vi "split columns.vi"(0 "Display string":string, 11 "error in":errorcluster) -> (4 "start chars":i32[](array[numeric]), 6 "Lengths":i32[](array[numeric]), 8 "Col Headers":string[](array[string]), 10 "Array":string[][](array[string]), 15 "error out":errorcluster)   [LabVIEW 2018]
uses:
  <vilib>/regexp/Match Regular Expression.xnode
panel:
  out "Display string 3":string
  out "Display string 2":string
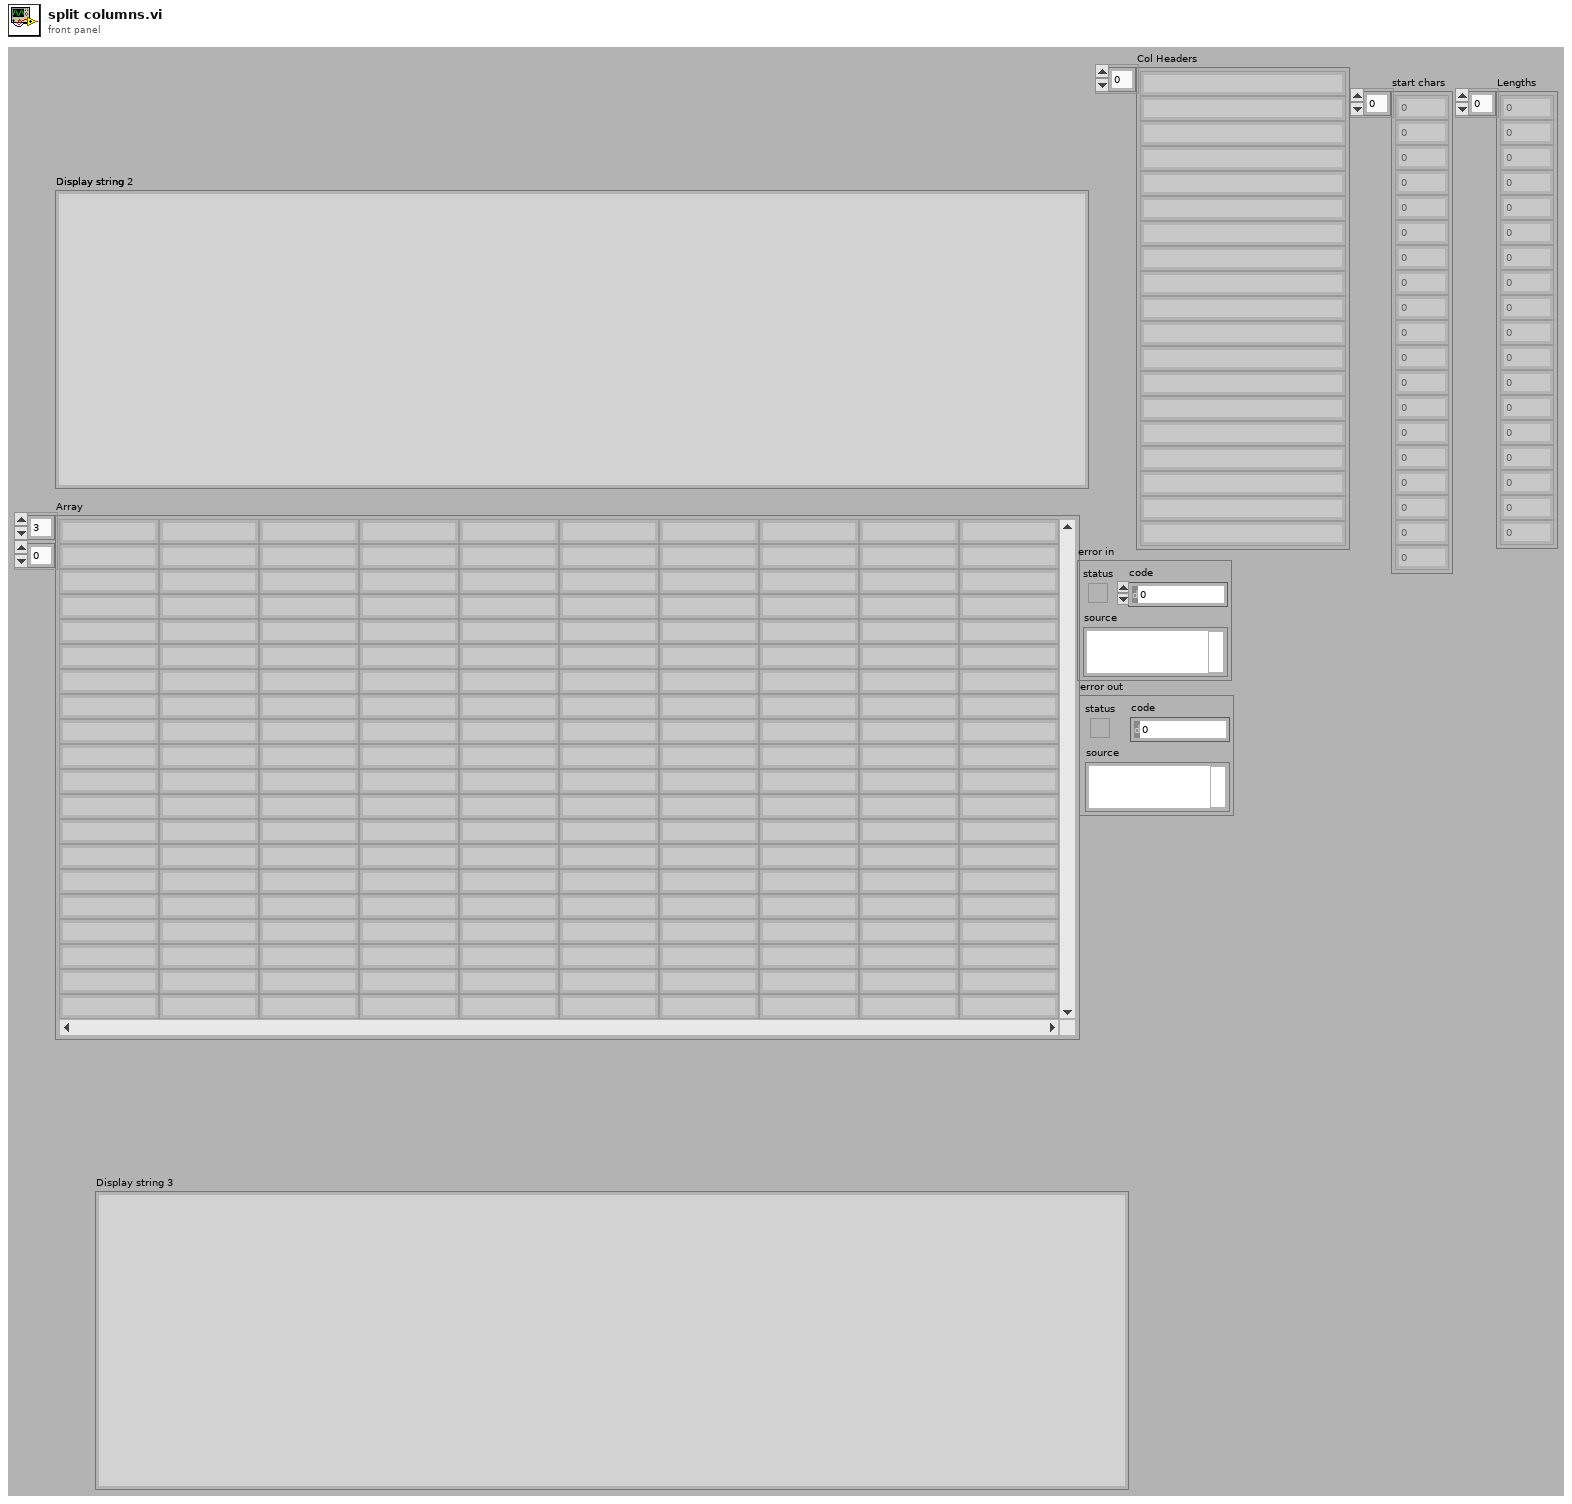
[diagram p1: front panel]
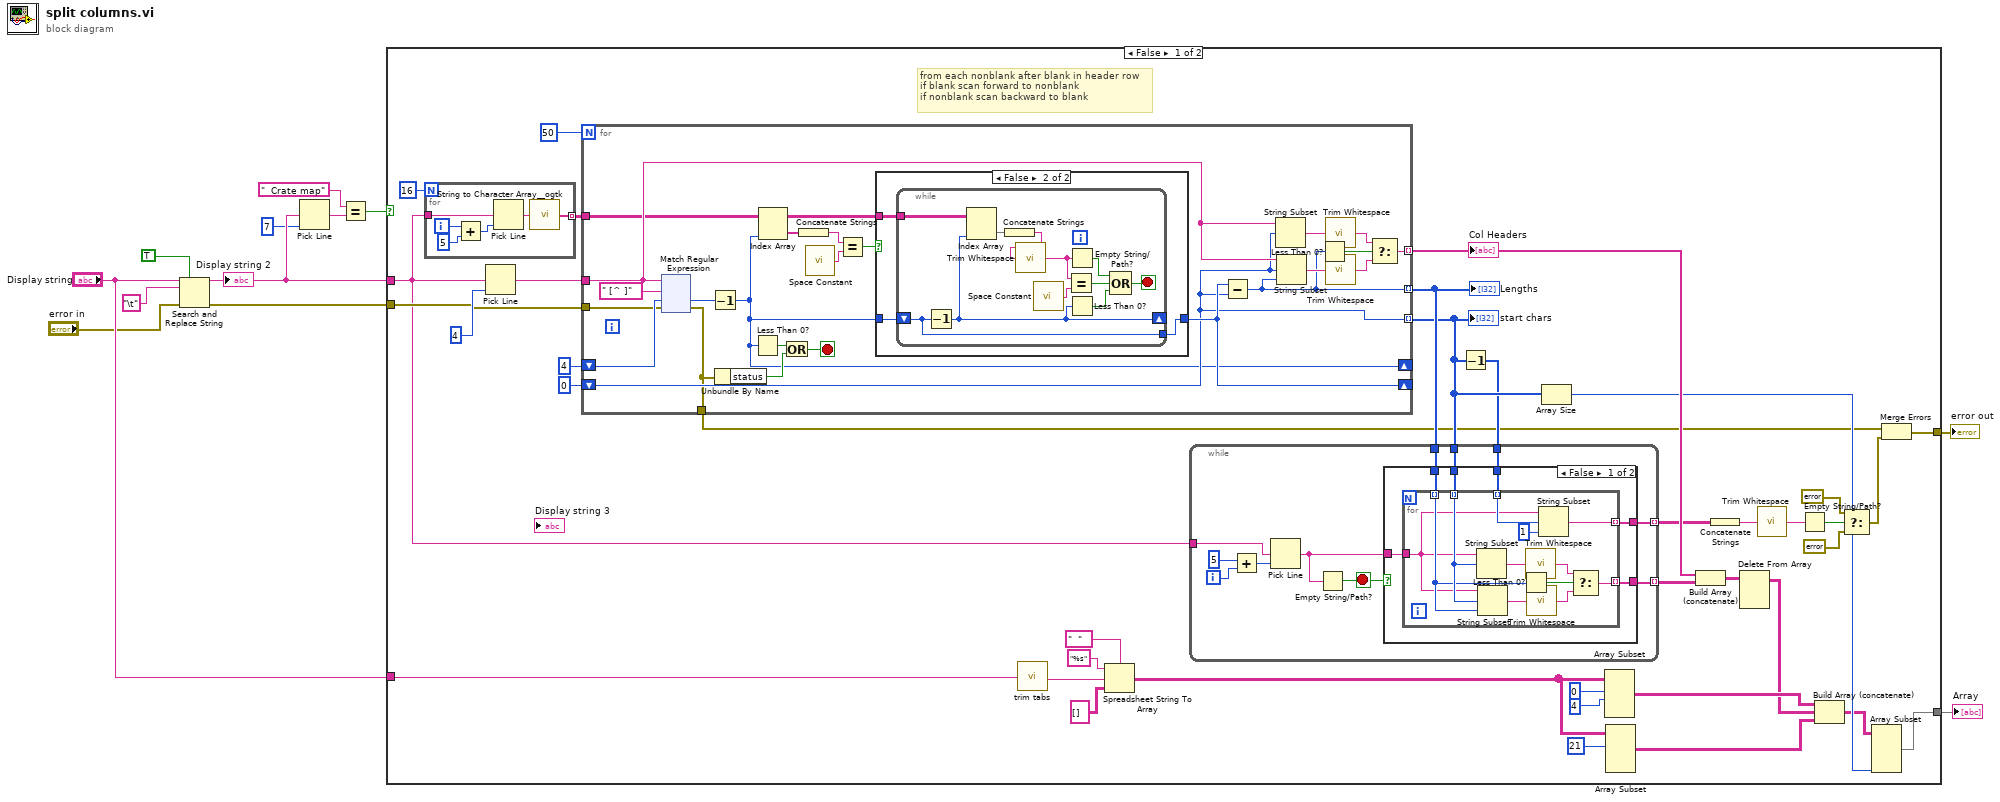
[diagram p0: block diagram]
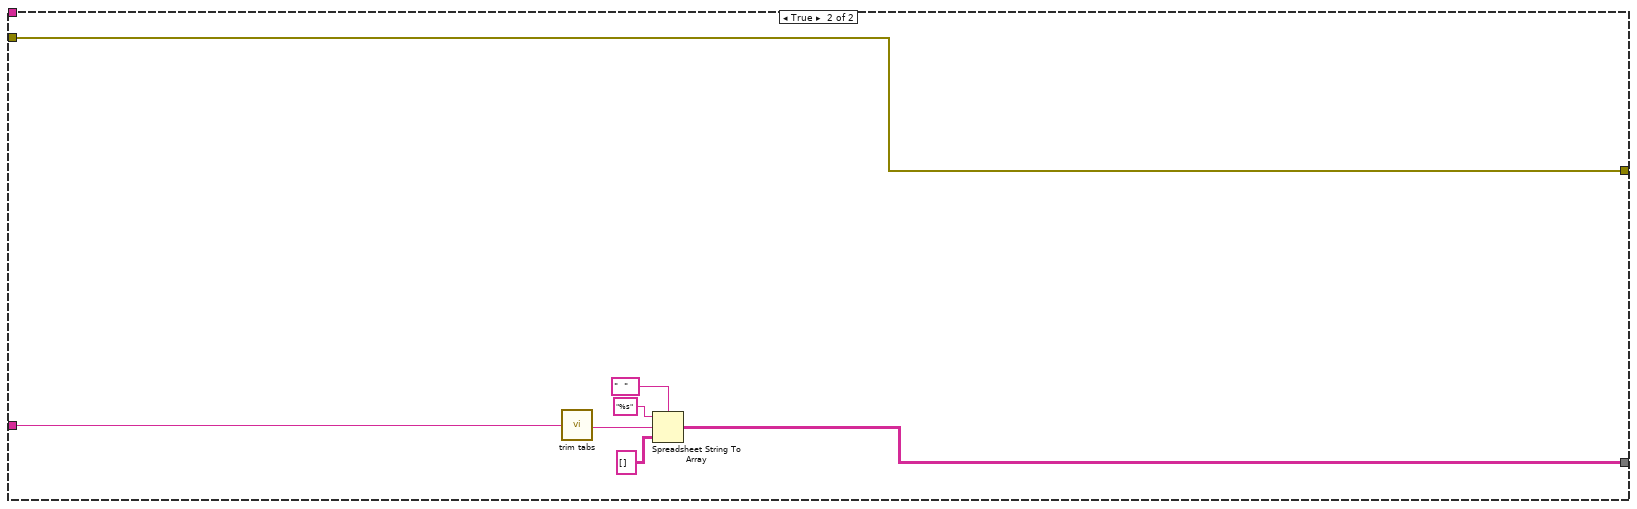
[diagram p4: hidden frame]
diagram:
  n1 = Search and Replace String(replace all?=TRUE ("replace all? (F)"), input string="Display string", search string="\t", error in="error in") -> (result string=w9:string, error out=w2:errorcluster)  [unwired: 4 in, 2 out]
  "Display string 2" <- w9
  n2 = Pick Line(multi-line string=w9, line index=7 ("x")) -> (output string=w7:string)  [unwired: 1 in]
  n3 = Equal?(x="  Crate map" ("search string/char (-)"), y=w7) -> (x = y?=w4:bool)
  n4 = case shown="False" w4 {
    tunnel: "Display string" -> [w43 w239]
    tunnel: w9 -> [w26 _]
    tunnel: [w29 w238] -> w5
    tunnel: w2 -> [w28 w237]
    tunnel: [w14 w237] -> w1
    frame False {
      # "from each nonblank after blank in header row\nif blank scan forward to nonblank\nif nonblank scan backward to blank"
      n5 = for {
        N: 16 -> [_]
        tunnel: w26 -> [w57]
        tunnel: [w52] -> w24 mode=indexing
        i -> [w55]
        n6 = Add(x=w55, y=5 ("x")) -> (x+y=w56:i32)
        n7 = Pick Line(multi-line string=w57, line index=w56) -> (output string=w53:string)  [unwired: 1 in]
        n8 = call <userlib>:"String to Character Array__ogtk.vi"("Input String"=w53) -> ("Character Array"=w52:string[])
      }
      n9 = Pick Line(multi-line string=w26, line index=4 ("x")) -> (output string=w51:string)  [unwired: 1 in]
      n10 = for {
        N: 50 -> [_]
        tunnel: w51 -> [w74]
        shift-right: [w60] -> _
        shift-left: 4 ("x") -> [w76]
        tunnel: [w73] -> w23 mode=indexing
        shift-right: [w78] -> _
        shift-left: 0 ("x") -> [w73]
        tunnel: [w67] -> w47 mode=indexing
        tunnel: [w71] -> w46 mode=indexing
        tunnel: w28 -> [w66]
        tunnel: [w63] -> w13
        tunnel: w24 -> [w61]
        stop <- w62 stop-if-true
        n11 = xnode "Match Regular Expression"("input string"=w74, "regular expression"=" [^ ]" ("search string/char (-)"), "offset (0)"=w76, "error in"=w66) -> ("offset past match"=w77:i32, "error out"=w63:errorcluster)  [unwired: 2 in, 3 out]
        n12 = Decrement(x=w77) -> (x-1=w60:i32)
        n13 = Unbundle By Name(w63) -> ("status"=w65:bool)
        n14 = Less Than 0?(x=w60) -> (x < 0?=w64:bool)
        n15 = Index Array(array=w61, index (col)=w60) -> (element=w59:string[])  [unwired: 1 in]
        n16 = Or(x=w64, y=w65) -> (x .or. y?=w62:bool)
        n17 = Concatenate Strings(w59) -> (w58:string)
        n18 = call <vilib>:"Space Constant.vi"() -> ("String"=w80:string)
        n19 = Equal?(x=w58, y=w80) -> (x = y?=w79:bool)
        n20 = case shown="False" w79 {
          tunnel: w60 -> [w193 w196]
          tunnel: [w193 w195] -> w78
          tunnel: w61 -> [_ w194]
          frame True {
          }
          frame False {
            n21 = while {
              shift-right: [w200] -> _
              shift-left: w196 -> [w206]
              tunnel: [w206] -> w195
              tunnel: w194 -> [w201]
              stop <- w203 stop-if-true
              n22 = Decrement(x=w206) -> (x-1=w200:i32)
              n23 = Index Array(array=w201, index (col)=w200) -> (element=w199:string[])  [unwired: 1 in]
              n24 = Concatenate Strings(w199) -> (w197:string)
              n25 = call <vilib>:"Trim Whitespace.vi"("string"=w197) -> ("trimmed string"=w198:string)  [unwired: 1 in]
              n26 = call <vilib>:"Space Constant.vi"() -> ("String"=w207:string)
              n27 = Equal?(x=w198, y=w207) -> (x = y?=w204:bool)
              n28 = Empty String/Path?(string/path=w198) -> (empty?=w205:bool)
              n29 = Less Than 0?(x=w200) -> (x < 0?=w202:bool)
              n30 = Compound Arithmetic op=OR(w205, w204, w202) -> (w203:bool)
            }
          }
        }
        n31 = Subtract(x=w78, y=w73) -> (x-y=w71:i32)
        n32 = String Subset(string=w74, offset (0)=w73) -> (substring=w72:string)  [unwired: 1 in]
        n33 = String Subset(string=w74, offset (0)=w73, length (rest)=w71) -> (substring=w75:string)
        n34 = Less Than 0?(x=w71) -> (x < 0?=w69:bool)
        n35 = call <vilib>:"Trim Whitespace.vi"("string"=w72) -> ("trimmed string"=w70:string)  [unwired: 1 in]
        n36 = call <vilib>:"Trim Whitespace.vi"("string"=w75) -> ("trimmed string"=w68:string)  [unwired: 1 in]
        n37 = Select(t=w70, s=w69, f=w68) -> (s? t:f=w67:string)
      }
      "Col Headers" <- w47
      "start chars" <- w23
      "Lengths" <- w46
      n38 = call "trim tabs.vi"("string"=w43) -> ("result string"=w42:string)
      n39 = Spreadsheet String To Array(delimiter (Tab)="  ", format string="%s" ("delimiter (Tab)"), spreadsheet string=w42, array type (2D Dbl)=string[][] [] ("appended array")) -> (array=w33:string[][])
      n40 = Decrement(x=w23) -> (x-1=w22:i32[])
      n41 = while {
        tunnel: w26 -> [w215]
        tunnel: w23 -> [w214]
        tunnel: w46 -> [w213]
        tunnel: [w212] -> w45 mode=indexing
        tunnel: w22 -> [w209]
        tunnel: [w208] -> w21 mode=indexing
        i -> [w216]
        stop <- w210 stop-if-true
        n42 = Add(x=5, y=w216) -> (x+y=w218:i32)
        n43 = Pick Line(multi-line string=w215, line index=w218) -> (output string=w211:string)  [unwired: 1 in]
        n44 = Empty String/Path?(string/path=w211) -> (empty?=w210:bool)
        n45 = case shown="False" w210 {
          tunnel: w214 -> [w224 _]
          tunnel: w213 -> [w223 _]
          tunnel: [w222 _] -> w212
          tunnel: w211 -> [w221 _]
          tunnel: w209 -> [w220 _]
          tunnel: [w219 _] -> w208
          frame False {
            n46 = for {
              tunnel: w221 -> [w226]
              tunnel: w224 -> [w230] mode=indexing
              tunnel: w223 -> [w229] mode=indexing
              tunnel: [w231] -> w222 mode=indexing
              tunnel: w220 -> [w228] mode=indexing
              tunnel: [w225] -> w219 mode=indexing
              n47 = String Subset(string=w226, offset (0)=w230) -> (substring=w233:string)  [unwired: 1 in]
              n48 = String Subset(string=w226, offset (0)=w230, length (rest)=w229) -> (substring=w232:string)
              n49 = Less Than 0?(x=w229) -> (x < 0?=w235:bool)
              n50 = call <vilib>:"Trim Whitespace.vi"("string"=w233) -> ("trimmed string"=w234:string)  [unwired: 1 in]
              n51 = call <vilib>:"Trim Whitespace.vi"("string"=w232) -> ("trimmed string"=w236:string)  [unwired: 1 in]
              n52 = String Subset(string=w226, offset (0)=w228, length (rest)=1 ("length (rest)")) -> (substring=w225:string)
              n53 = Select(t=w234, s=w235, f=w236) -> (s? t:f=w231:string)
            }
          }
          frame True {
          }
        }
      }
      n54 = Array Size(array=w23) -> (size(s)=w31:i32)
      n55 = Array Subset(array=w33, index (row)=0 ("index"), length (row)=4 ("index")) -> (w35:string[][])  [unwired: 2 in]
      n56 = Array Subset(array=w33, index (row)=21 ("index")) -> (w34:string[][])  [unwired: 3 in]
      n57 = Build Array (concatenate)(w47, w45) -> (w44:string[][])
      n58 = Concatenate Strings(w21) -> (w20:string)
      n59 = Delete From Array(array=w44) -> (array with subset deleted=w32:string[][])  [unwired: 3 in, 1 out]
      n60 = call <vilib>:"Trim Whitespace.vi"("string"=w20) -> ("trimmed string"=w19:string)  [unwired: 1 in]
      n61 = Empty String/Path?(string/path=w19) -> (empty?=w18:bool)
      n62 = Build Array (concatenate)(w35, w32, w34) -> (w30:string[][])
      n63 = Select(t=errorcluster {"status"=FALSE, "code"=0, "source"=""}, s=w18, f=errorcluster {"status"=TRUE, "code"=0, "source"="Overlapping columns!"} ("error out")) -> (s? t:f=w15:errorcluster)
      n64 = Array Subset(array=w30, length (col)=w31) -> (w29:string[][])  [unwired: 3 in]
      n65 = Merge Errors(w13, w15) -> (w14:errorcluster)
    }
    frame True {
      n66 = call "trim tabs.vi"("string"=w239) -> ("result string"=w243:string)
      n67 = Spreadsheet String To Array(delimiter (Tab)="  ", format string="%s" ("delimiter (Tab)"), spreadsheet string=w243, array type (2D Dbl)=string[][] [] ("appended array")) -> (array=w238:string[][])
    }
  }
  "Array" <- w5
  "error out" <- w1
